vi "fmt_formatTimeColumn.vi"(4 "channel index":i32, 6 "length":i32, 7 "styles map":string[](array[string]), 8 "error in (no error)":errorcluster, 9 "dt":dbl=1.0, 10 "t0":timestamp, 11 "format buffers in":T1) -> (0 "error out":errorcluster, 2 "data column index":i32, 3 "format buffers out":T1)   [LabVIEW 2020, in "NI_ExcelFile.lvlib"]
uses:
  <vilib>/express/express shared/NI_ExcelFile/NI_ExcelFile.lvlib
  <vilib>/express/express shared/NI_ExcelFile/Ctrls/fmt_formatBuffer.ctl
  <vilib>/express/express shared/NI_ExcelFile/Ctrls/TimeColumnMode.ctl
  <vilib>/express/express shared/NI_ExcelFile/Ctrls/Columns.ctl
  <vilib>/express/express shared/NI_ExcelFile/Ctrls/ColumnInfo.ctl
  <vilib>/express/express shared/NI_ExcelFile/Ctrls/DataType.ctl
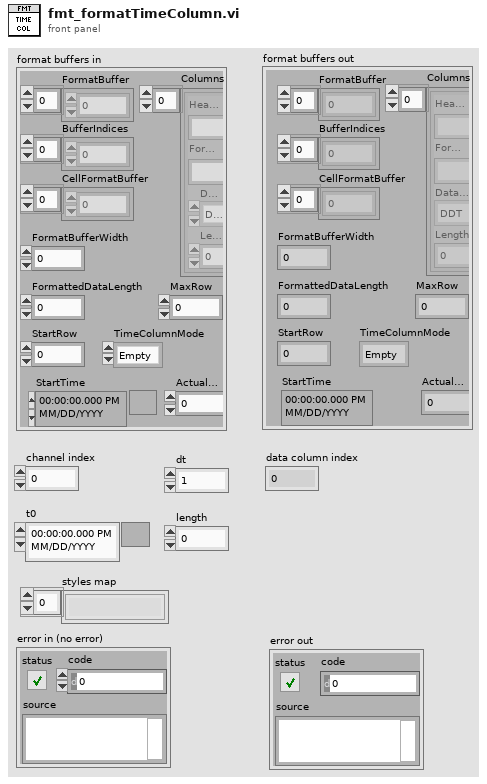
[diagram p1: front panel]
types:
  T1 = typedef "NI_ExcelFile.lvlib/fmt_formatBuffer.ctl" = cluster{"FormatBuffer":u8[], "BufferIndices":i32[], "CellFormatBuffer":u8[], "FormatBufferWidth":i32, "FormattedDataLength":i32, "MaxRow":i32, "StartRow":i32, "TimeColumnMode":T2, "StartTime":timestamp, "Columns":T3, "ActualLength":i32}
  T2 = typedef "NI_ExcelFile.lvlib/TimeColumnMode.ctl" = enum16{"Empty", "OnePerCh", "One"}
  T3 = typedef "NI_ExcelFile.lvlib/Columns.ctl" = T4[]
  T4 = typedef "NI_ExcelFile.lvlib/ColumnInfo.ctl" = cluster{"Header":string, "Format":string, "DataType":T5, "Length":u64}
  T5 = typedef "NI_ExcelFile.lvlib/DataType.ctl" = enum16{"DDT", "WFM", "Array of STR", "Array of DBL", "Array of I8", "Array of I16", "Array of I32", "Array of I64", "Array of SGL", "Array of U8", "Array of U16", "Array of U32", "Array of U64", "Array of Time"}
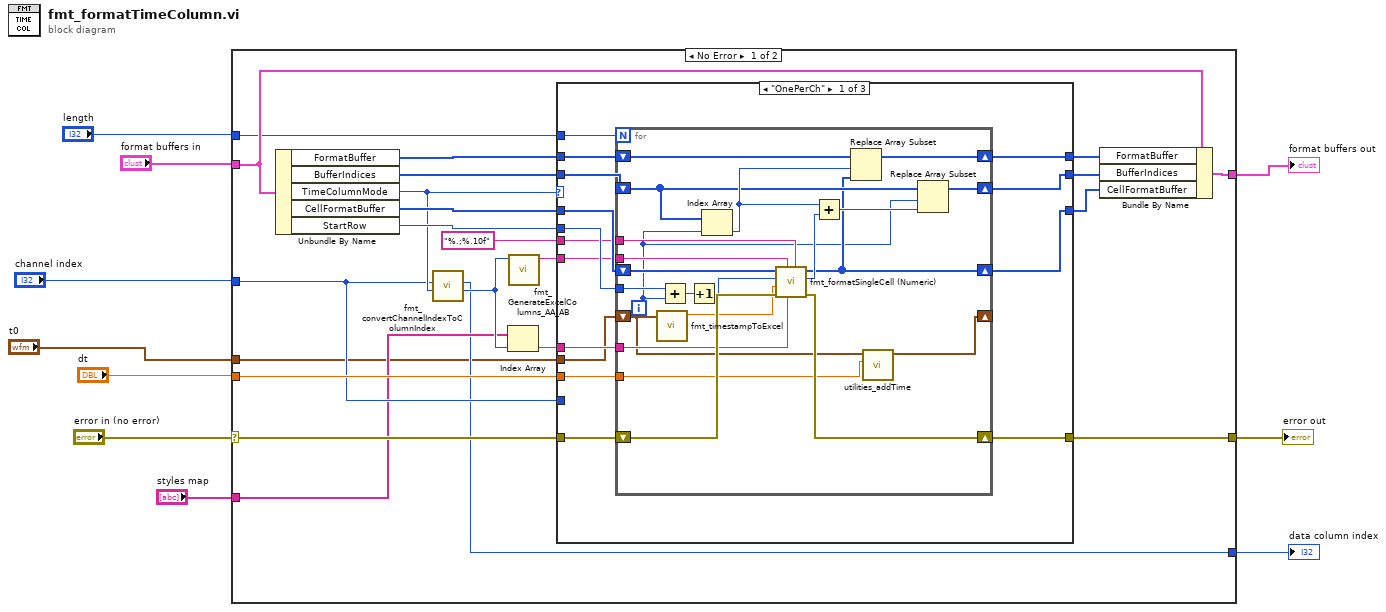
[diagram p0: block diagram]
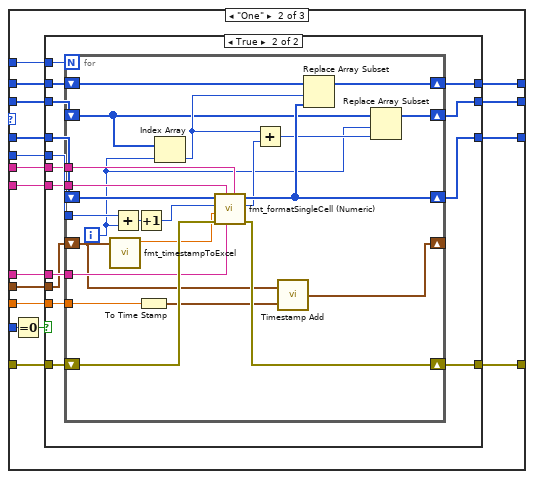
[diagram p2: hidden frame]
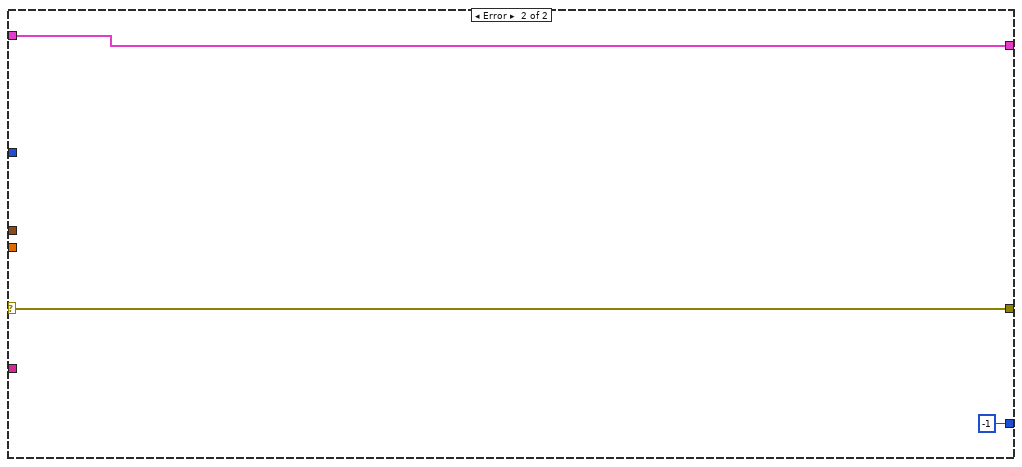
[diagram p5: hidden frame]
diagram:
  n1 = case shown="No Error" "error in (no error)" {
    selector: "error in (no error)" -> [w19 w134]
    tunnel: [w32 w135] -> w10
    tunnel: "format buffers in" -> [w31 w135]
    tunnel: "channel index" -> [w20 _]
    tunnel: "length" -> [w26 _]
    tunnel: "t0" -> [w11 _]
    tunnel: "dt" -> [w25 _]
    tunnel: [w18 w134] -> w3
    tunnel: "styles map" -> [w14 _]
    tunnel: [w12 -1 ("data column index")] -> w1
    frame No Error {
      n2 = Unbundle By Name(w31) -> ("FormatBuffer"=w30:u8[], "BufferIndices"=w28:i32[], "TimeColumnMode"=w21:T2, "CellFormatBuffer"=w24:u8[], "StartRow"=w22:i32)
      n3 = call <vilib>:"fmt_convertChannelIndexToColumnIndex.vi"("TimeColumnMode"=w21, "channel index"=w20) -> ("time column index"=w15:i32, "data column index"=w12:i32)  [unwired: 8 in]
      n4 = Index Array(array=w14, index=w15) -> (element=w13:string)
      n5 = call <vilib>:"fmt_GenerateExcelColumns_AA_AB.vi"("NumColumns"=w15) -> ("Column"=w17:string)  [unwired: 10 in]
      n6 = case shown="\"OnePerCh\"" w21 {
        tunnel: w30 -> [w42 w83 w132]
        tunnel: [w46 w84 w132] -> w29
        tunnel: w28 -> [w41 w81 w131]
        tunnel: [w45 w82 w131] -> w27
        tunnel: w20 -> [_ w86 _]
        tunnel: w26 -> [w47 w80 _]
        tunnel: w11 -> [w33 w79 _]
        tunnel: w25 -> [w43 w78 _]
        tunnel: w24 -> [w40 w77 w130]
        tunnel: [w44 w76 w130] -> w23
        tunnel: w22 -> [w39 w75 _]
        tunnel: w19 -> [w37 w74 w129]
        tunnel: [w38 w73 w129] -> w18
        tunnel: w17 -> [w36 w72 _]
        tunnel: "%.;%.10f" ("format string") -> [w35 w71 _]
        tunnel: w13 -> [w34 w70 _]
        frame "OnePerCh" {
          n7 = for {
            N: w47 -> [_]
            shift-right: [w65] -> w46
            shift-left: w42 -> [w66]
            shift-right: [w62] -> w45
            shift-left: w41 -> [w61]
            tunnel: w43 -> [w48]
            shift-right: [w56] -> w44
            shift-left: w40 -> [w69]
            tunnel: w39 -> [w68]
            shift-right: [w58] -> w38
            shift-left: w37 -> [w59]
            tunnel: w36 -> [w57]
            tunnel: w35 -> [w54]
            tunnel: w34 -> [w53]
            shift-right: [w50] -> _
            shift-left: w33 -> [w51]
            i -> [w52]
            n8 = call <vilib>:"fmt_timestampToExcel.vi"("timestamp"=w51) -> ("Excel timestamp"=w49:dbl)  [unwired: 10 in]
            n9 = Add(x=w68, y=w52) -> (x+y=w67:i32)
            n10 = Increment(x=w67) -> (x+1=w55:i32)
            n11 = Index Array(array=w61, index=w52) -> (element=w64:i32)
            n12 = call <vilib>:"fmt_formatSingleCell (Numeric).vi"("format string"=w54, "style index"=w53, "Column"=w57, "error in"=w59, "Value"=w49, "Row"=w55, "Format buffer"=w69) -> ("error out"=w58:errorcluster, "Buffer size"=w63:i32, "Formatted buffer"=w56:u8[])  [unwired: 1 in, 1 out]
            n13 = Add(x=w64, y=w63) -> (x+y=w60:i32)
            n14 = Replace Array Subset(array=w66, new element=w56, index=w64) -> (w65:u8[])
            n15 = call <vilib>:"utilities_addTime.vi"("number"=w48, "Time"=w51) -> ("Time out"=w50:timestamp)  [unwired: 9 in]
            n16 = Replace Array Subset(array=w61, new element=w60, index=w52) -> (w62:i32[])
          }
        }
        frame "One" {
          n17 = Equal To 0?(x=w86) -> (x = 0?=w85:bool)
          n18 = case shown="True" w85 {
            tunnel: [w90 w105] -> w84
            tunnel: w83 -> [w90 w104]
            tunnel: [w89 w103] -> w82
            tunnel: w81 -> [w89 w102]
            tunnel: w80 -> [_ w101]
            tunnel: w79 -> [_ w91]
            tunnel: w78 -> [_ w100]
            tunnel: w77 -> [w88 w99]
            tunnel: [w88 w98] -> w76
            tunnel: w75 -> [_ w97]
            tunnel: w74 -> [w87 w96]
            tunnel: [w87 w95] -> w73
            tunnel: w72 -> [_ w94]
            tunnel: w71 -> [_ w93]
            tunnel: w70 -> [_ w92]
            frame False {
            }
            frame True {
              n19 = for {
                N: w101 -> [_]
                shift-right: [w124] -> w105
                shift-left: w104 -> [w125]
                shift-right: [w120] -> w103
                shift-left: w102 -> [w119]
                tunnel: w100 -> [w110]
                shift-right: [w123] -> w98
                shift-left: w99 -> [w128]
                tunnel: w97 -> [w127]
                shift-right: [w116] -> w95
                shift-left: w96 -> [w117]
                tunnel: w94 -> [w115]
                tunnel: w93 -> [w114]
                tunnel: w92 -> [w112]
                shift-right: [w106] -> _
                shift-left: w91 -> [w107]
                i -> [w111]
                n20 = call <vilib>:"fmt_timestampToExcel.vi"("timestamp"=w107) -> ("Excel timestamp"=w109:dbl)  [unwired: 10 in]
                n21 = Add(x=w127, y=w111) -> (x+y=w126:i32)
                n22 = Increment(x=w126) -> (x+1=w113:i32)
                n23 = To Time Stamp(1:w110) -> (0:w108:timestamp)
                n24 = Index Array(array=w119, index=w111) -> (element=w122:i32)
                n25 = call <vilib>:"fmt_formatSingleCell (Numeric).vi"("format string"=w114, "style index"=w112, "Column"=w115, "error in"=w117, "Value"=w109, "Row"=w113, "Format buffer"=w128) -> ("error out"=w116:errorcluster, "Buffer size"=w121:i32, "Formatted buffer"=w123:u8[])  [unwired: 1 in, 1 out]
                n26 = Add(x=w122, y=w121) -> (x+y=w118:i32)
                n27 = call <vilib>:"Timestamp Add.vi"("y"=w108, "x"=w107) -> ("x + y"=w106:timestamp)
                n28 = Replace Array Subset(array=w125, new element=w123, index=w122) -> (w124:u8[])
                n29 = Replace Array Subset(array=w119, new element=w118, index=w111) -> (w120:i32[])
              }
            }
          }
        }
        frame "Empty", Default {
        }
      }
      n30 = Bundle By Name(cluster=w31, "FormatBuffer"=w29, "BufferIndices"=w27, "CellFormatBuffer"=w23) -> (w32:T1)
    }
    frame Error {
    }
  }
  "format buffers out" <- w10
  "error out" <- w3
  "data column index" <- w1
